vi "Check Format String.vi"(8 "error in (no error)":errorcluster, 11 "format string in":string) -> (0 "error out":errorcluster, 2 "# of format strings":i32, 3 "format string out":string)   [LabVIEW 2017]
uses:
  <vilib>/regexp/Match Regular Expression.xnode
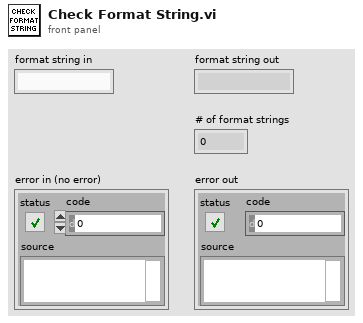
[diagram p1: front panel]
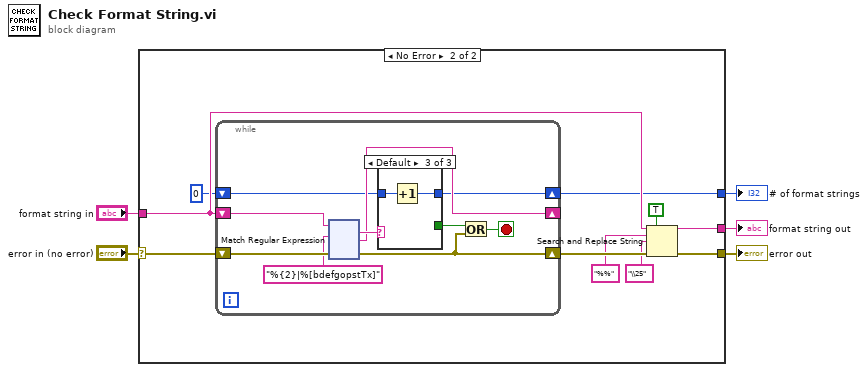
[diagram p0: block diagram]
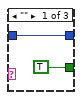
[diagram p3: hidden frame]
diagram:
  n1 = case shown="No Error" "error in (no error)" {
    selector: "error in (no error)" -> [w6 w7]
    tunnel: "format string in" -> [_ w15]
    tunnel: [_ w11] -> w4
    tunnel: [_ w9] -> w3
    tunnel: [w6 w8] -> w1
    frame Error {
    }
    frame No Error {
      n2 = while {
        shift-right: [w22] -> _
        shift-left: w15 -> [w23]
        shift-right: [w20] -> w9
        shift-left: 0 ("size(s)") -> [w21]
        shift-right: [w18] -> w16
        shift-left: w7 -> [w26]
        stop <- w17 stop-if-true
        n3 = xnode "Match Regular Expression"("input string"=w23, "regular expression"="%{2}|%[bdefgopstTx]", "error in"=w26) -> ("whole match"=w25:string, "after match"=w22:string, "error out"=w18:errorcluster)  [unwired: 3 in, 2 out]
        n4 = case shown="Default" w25 {
          tunnel: [TRUE _ _] -> w19
          tunnel: w21 -> [w27 w29 w31]
          tunnel: [w27 w29 w30] -> w20
          frame "" {
          }
          frame "%%" {
          }
          frame Default {
            n5 = Increment(x=w31) -> (x+1=w30:i32)
          }
        }
        n6 = Or(x=w19, y=w18) -> (x .or. y?=w17:bool)
      }
      n7 = Search and Replace String(replace all?=TRUE ("replace all? (F)"), input string=w15, search string="%%", replace string="\\25" ("replace string (\"\")"), error in=w16) -> (result string=w11:string, error out=w8:errorcluster)  [unwired: 3 in, 2 out]
    }
  }
  "format string out" <- w4
  "# of format strings" <- w3
  "error out" <- w1
